vi "Restore Configuration.vi"(8 "error in (no error)":errorcluster, 9 "Initialization":bool, 10 "File path":path, 11 "Measure Object in":refnum<class "Template Module.lvclass">) -> (0 "error out":errorcluster, 1 "Section out":string, 2 "File path out":path, 3 "Measure Object out":refnum<class "Template Module.lvclass">)   [LabVIEW 2021, in "Template Module.lvclass"]
uses:
  Template Module.lvclass
  Template Module.lvclass/Template Module.ctl
  Read Name.vi
  Template Module Messages/Restore Configuration Msg/Restore Configuration Msg.lvclass
panel:
  out "Numeric":i32
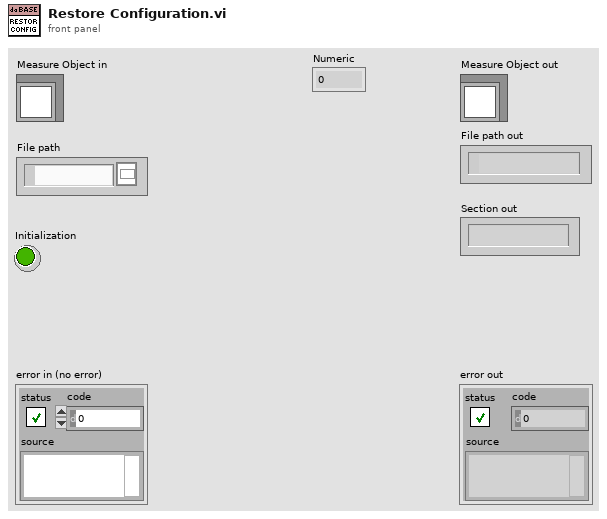
[diagram p1: front panel]
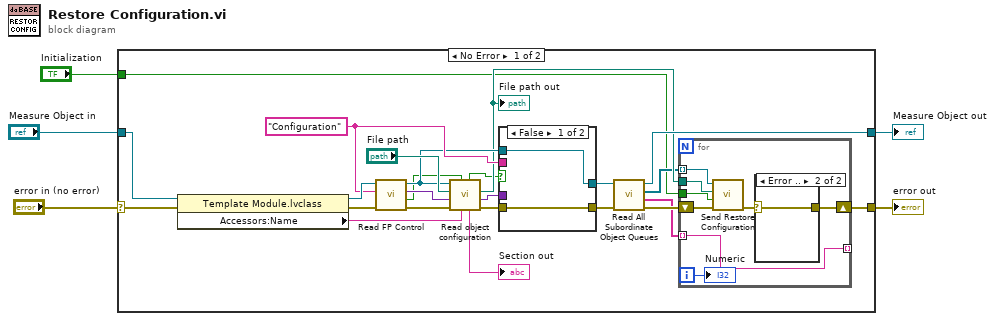
[diagram p0: block diagram]
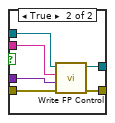
[diagram p2: hidden frame]
diagram:
  n1 = case shown="No Error" "error in (no error)" {
    selector: "error in (no error)" -> [w25 w49]
    tunnel: [w11 w49] -> w4
    tunnel: [w15 w48] -> w2
    tunnel: "Measure Object in" -> [w24 w48]
    tunnel: "Initialization" -> [w7 _]
    frame No Error {
      w21 = "Configuration" ("Control Name")
      n2 = property class="Template Module.lvclass"(reference=w24, error in=w25) -> (reference out=w23:refnum<class "Template Module.lvclass">, error out=w26:errorcluster, "Accessors:Name"=w22:string)
      n3 = call-dynamic "Read FP Control.vi"("error in (no error)"=w26, "Control Name"=w21, "Measure Object in"=w23) -> ("error out"=w27:errorcluster, "Present"=w8:bool, "Control Value"=w29:variant, "Measure Object out"=w18:refnum<class "Template Module.lvclass">)  [unwired: 5 in]
      n4 = call "Read object configuration.vi"("Object name"=w22, "Present"=w8, "Error In"=w27, "type"=w29, "File path"="File path", "object"=w18) -> ("Error Out"=w19:errorcluster, "Configuration"=w20:variant, "File path out"=w14:path, "Section out"=→"Section out":string, "found?"=w9:bool)  [unwired: 1 in]
      "File path out" <- w14
      n5 = case shown="False" w9 {
        tunnel: w21 -> [_ w37]
        tunnel: w20 -> [_ w36]
        tunnel: w19 -> [w31 w35]
        tunnel: w18 -> [w30 w34]
        tunnel: [w31 w33] -> w17
        tunnel: [w30 w32] -> w16
        frame False {
        }
        frame True {
          n6 = call-dynamic "Write FP Control.vi"("error in (no error)"=w35, "Control Value"=w36, "Control Name"=w37, "Measure Object in"=w34) -> ("error out"=w33:errorcluster, "Measure Object out"=w32:refnum<class "Template Module.lvclass">)  [unwired: 6 in]
        }
      }
      n7 = call-dynamic "Read All Subordinate Object Queues.vi"("error in (no error)"=w17, "Measure Object in"=w16) -> ("error out"=w12:errorcluster, "Object names"=w6:string[], "Object enqueuers"=w13:refnum<class "Message Enqueuer.lvclass">[], "Measure Object out"=w15:refnum<class "Template Module.lvclass">)  [unwired: 6 in]
      n8 = for {
        tunnel: w14 -> [w45]
        tunnel: w13 -> [w44] mode=indexing
        shift-right: [w40] -> w11
        shift-left: w12 -> [w43]
        tunnel: w7 -> [w42]
        tunnel: w6 -> [w39] mode=indexing
        tunnel: [w39] -> _ mode=indexing
        i -> [w38]
        n9 = call "Send Restore Configuration.vi"("error in (no error)"=w43, "Initialization"=w42, "File path"=w45, "Message Enqueuer"=w44) -> ("error out"=w41:errorcluster)  [unwired: 6 in, 1 out]
        n10 = case shown="Error .." w41 {
          selector: w41 -> [w46 w47]
          tunnel: [w46 w47] -> w40
          frame No Error {
          }
          frame Error {
          }
        }
        "Numeric" <- w38
      }
    }
    frame Error {
    }
  }
  "error out" <- w4
  "Measure Object out" <- w2
